vi "Periodic Tasks.vi"(8 "error in":errorcluster) -> ()   [LabVIEW 2013]
doc: "This VI runs in parallel to other tasks. It can contain as many user-defined periodic loops as you need. These can carry out PID or other sorts of timed response."
uses:
  <vilib>/Rock Robotics/SystemInterfaces/Utilities/FPGA_UtilitiesLED Source.ctl
  <vilib>/Rock Robotics/SystemInterfaces/Utilities/FPGA_UtilitiesLED State.ctl
  <vilib>/Rock Robotics/WPI/DriverStation/DriverStationLCD/WPI_DriverStationLCDLCDLine.ctl
  Robot Global Data.vi
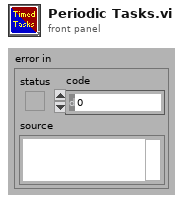
[diagram p1: front panel]
types:
  T1 = typedef "WPI_DigitalInputDevRef.ctl" = cluster{"DevStatus":errorcluster, "DIO Channel":T2, "Digital Module":T3}
  T2 = typedef "FPGA_DIOChannel.ctl" = enum8{"DIO 1", "DIO 2", "DIO 3", "DIO 4", "DIO 5", "DIO 6", "DIO 7", "DIO 8", "DIO 9", "DIO 10", "DIO 11", "DIO 12", "DIO 13", "DIO 14", "Invalid"}
  T3 = typedef "FPGA_TypedefDigitalModule.ctl" = enum16{"Digital Module 1", "Digital Module 2"}
  T4 = typedef "WPI_AnalogChannelDevRef.ctl" = cluster{"DevStatus":errorcluster, "Analog Module":T5, "Analog Channel":T6}
  T5 = typedef "FPGA_TypedefAnalogModule.ctl" = enum16{"Analog Module 1", "Analog Module 2"}
  T6 = typedef "FPGA_AIChannel.ctl" = enum8{"AI 1", "AI 2", "AI 3", "AI 4", "AI 5", "AI 6", "AI 7", "AI 8", "Invalid"}
  T7 = typedef "WPI_EncoderDevRef.ctl" = cluster{"DevStatus":errorcluster, "EncoderIndex":T8, "CounterIndex":T9, "DistancePerCount":dbl, "Decoding Type":T10}
  T8 = typedef "FPGA_EncoderIdx.ctl" = enum8{"Enc 0", "Enc 1", "Enc 2", "Enc 3", "Invalid"}
  T9 = typedef "FPGA_CounterCtrSystemIndex.ctl" = enum8{"Ctr 0", "Ctr 1", "Ctr 2", "Ctr 3", "Ctr 4", "Ctr 5", "Ctr 6", "Ctr 7", "Invalid"}
  T10 = typedef "WPI_EncoderType.ctl" = enum16{"1x", "2x", "4x"}
  T11 = cluster{"Winch Desired Location":dbl, "Winch Desired Location 2":dbl, "Winch Desired Location 3":dbl}
  T12 = typedef "FPGA_UtilitiesLED State.ctl" = enum16{"Off", "On", "Toggle"}
  T13 = typedef "FPGA_UtilitiesLED Source.ctl" = enum16{"User LED", "FPGA LED"}
  T14 = typedef "WPI_DriverStationLCDLCDLine.ctl" = enum16{"Main - Line 1", "User - Line 2", "User - Line 3", "User - Line 4", "User - Line 5", "User - Line 6"}
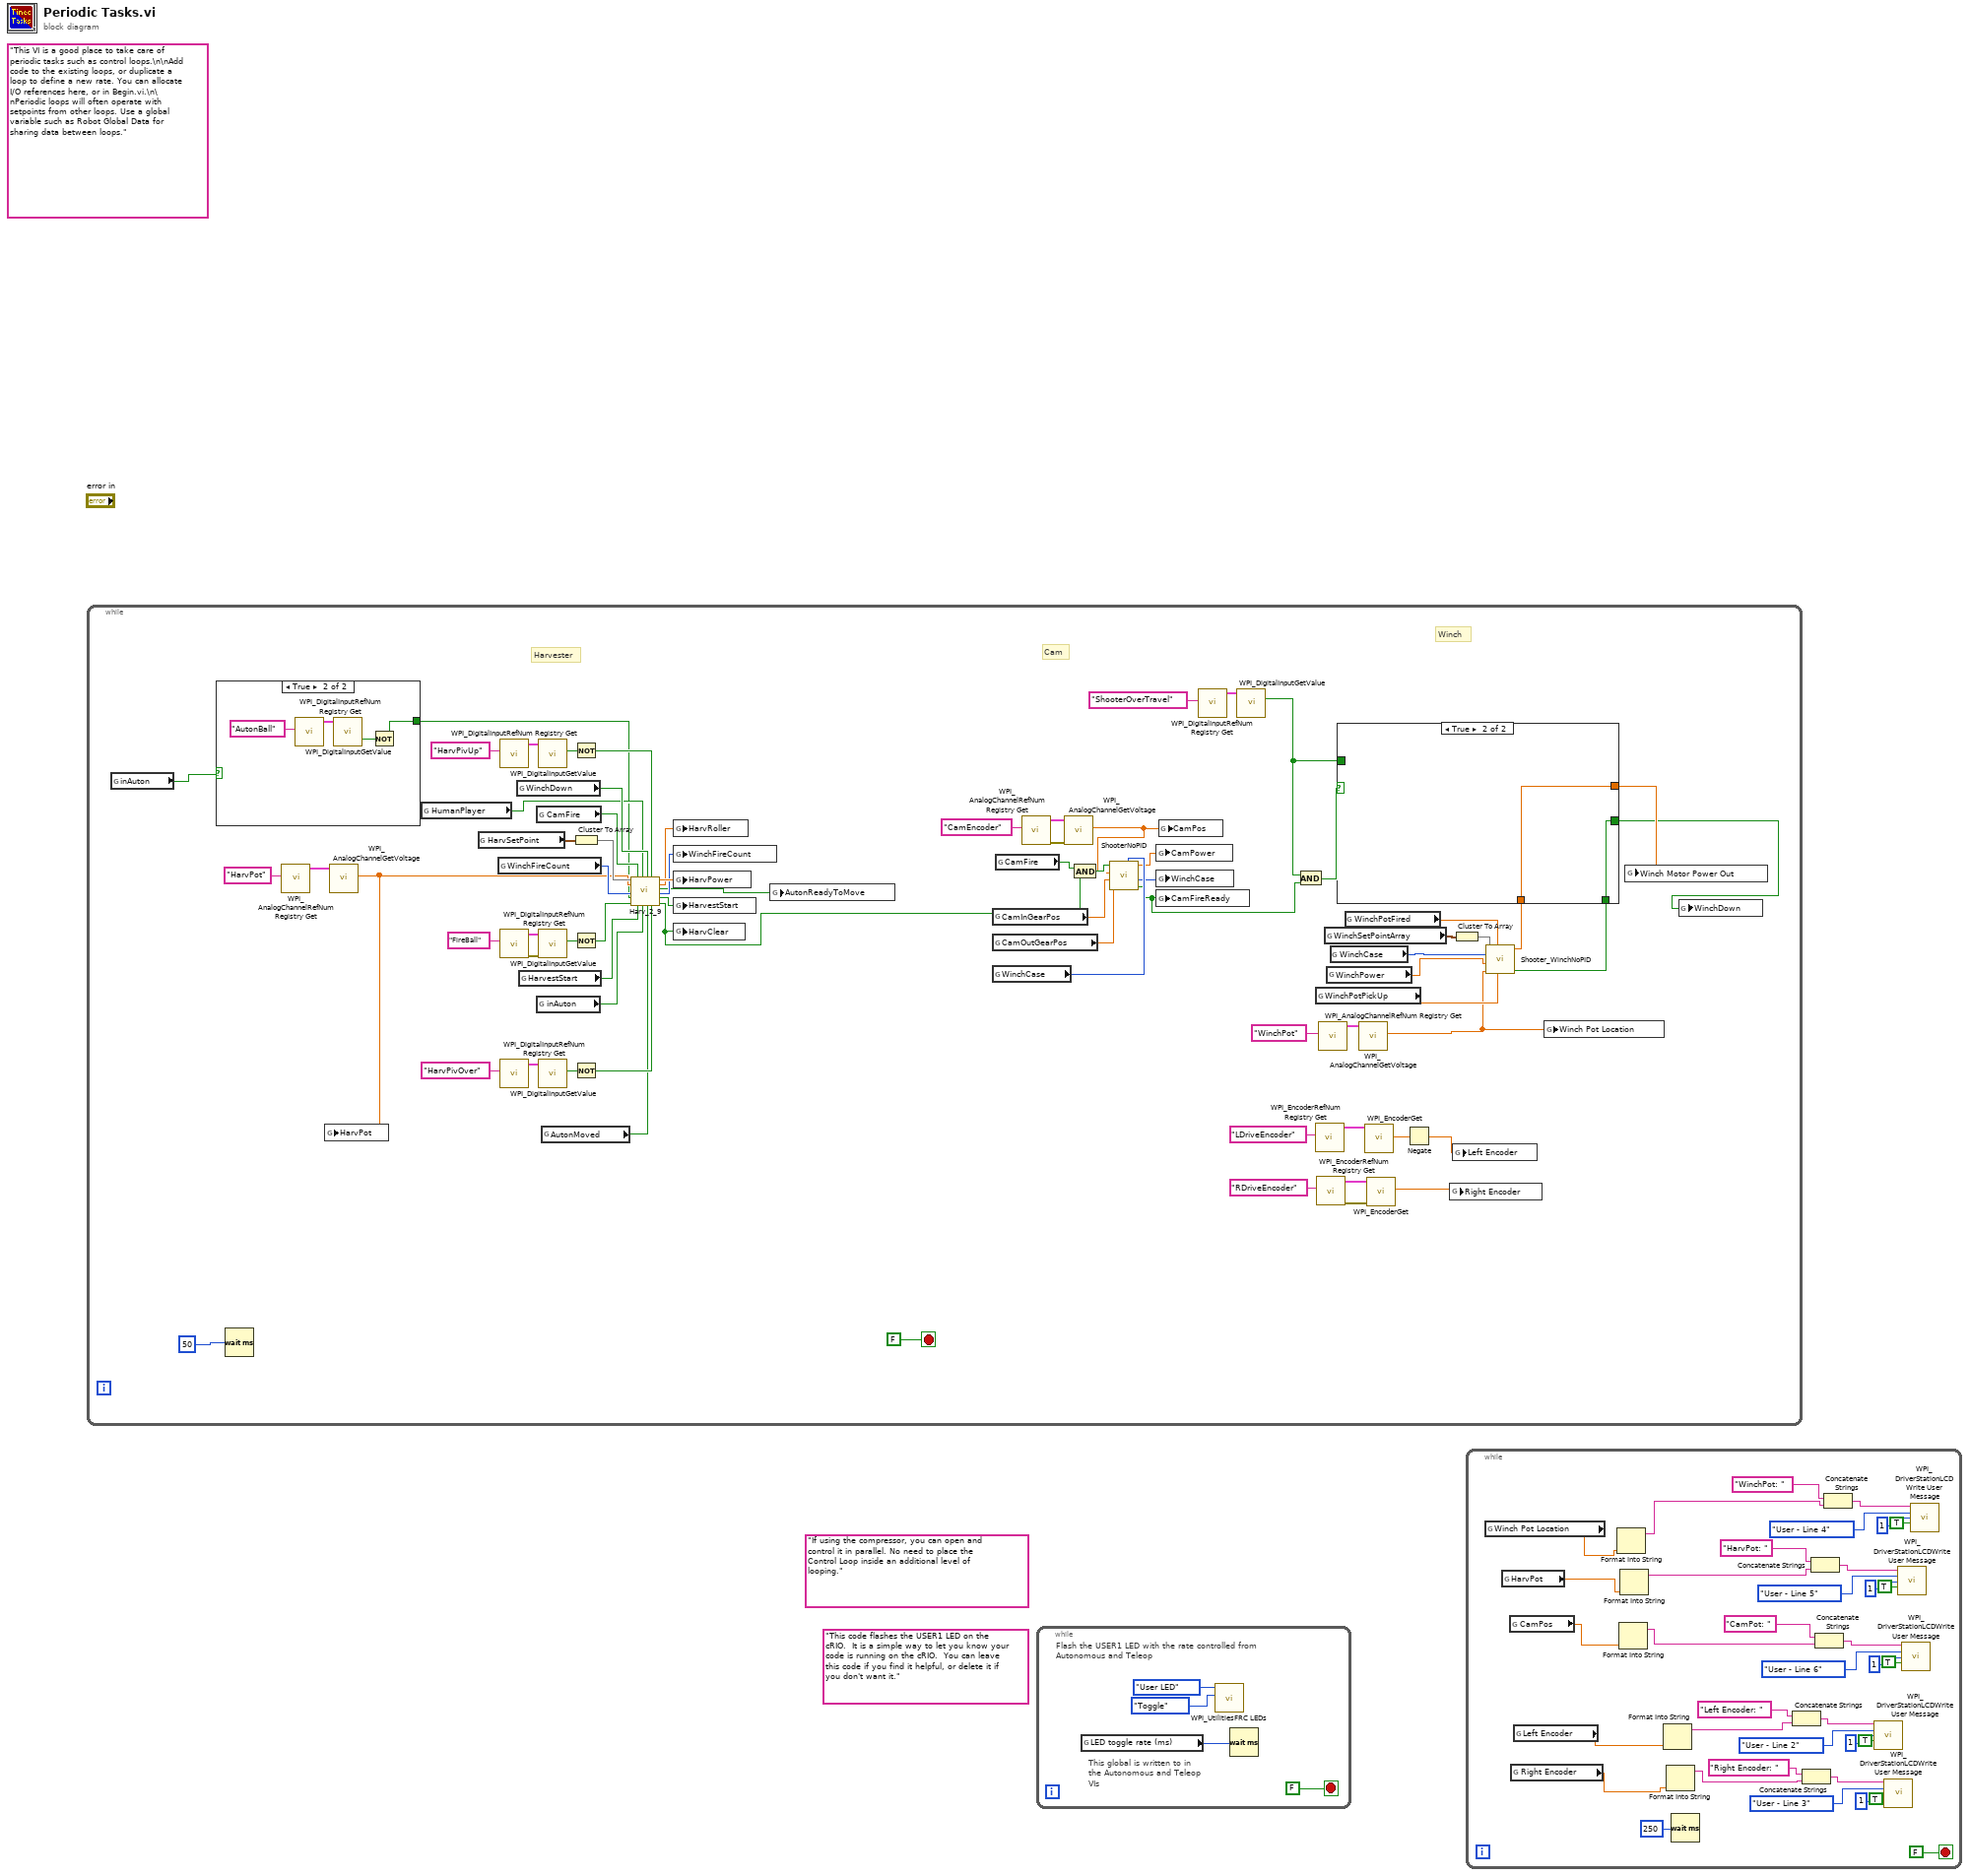
[diagram p0: block diagram]
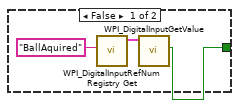
[diagram p2: hidden frame]
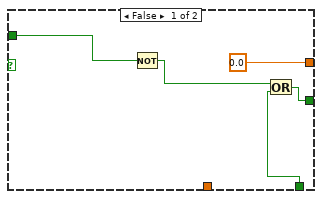
[diagram p3: hidden frame]
diagram:
  (unwired) "If using the compressor, you can open and control it in parallel. No need to place the Control Loop inside an additional level of looping."
  (unwired) "This code flashes the USER1 LED on the cRIO.  It is a simple way to let you know your code is running on the cRIO.  You can leave this code if you find it helpful, or delete it if you don't want it."
  (unwired) "This VI is a good place to take care of periodic tasks such as control loops.\n\nAdd code to the existing loops, or duplicate a loop to define a new rate. You can allocate I/O references here, or in Begin.vi.\n\nPeriodic loops will often operate with setpoints from other loops. Use a global variable such as Robot Global Data for sharing data between loops."
  n1 = while {
    stop <- FALSE stop-if-true
    # "Winch"
    # "Cam"
    # "Harvester"
    n2 = global read "Robot Global Data.vi" "inAuton"() -> (w2:bool)
    n3 = case shown="True" w2 {
      tunnel: [w73 w77] -> w1
      frame False {
        n4 = call <vilib>:"WPI_DigitalInputRefNum Registry Get.vi"("refnum name"="BallAquired") -> ("DigitalInputDevRef"=w75:T1)  [unwired: 9 in, 1 out]
        n5 = call <vilib>:"WPI_DigitalInputGetValue.vi"("DigitalInputDevRef"=w75) -> ("Value"=w73:bool)  [unwired: 8 in, 2 out]
      }
      frame True {
        n6 = call <vilib>:"WPI_DigitalInputRefNum Registry Get.vi"("refnum name"="AutonBall") -> ("DigitalInputDevRef"=w79:T1)  [unwired: 9 in, 1 out]
        n7 = call <vilib>:"WPI_DigitalInputGetValue.vi"("DigitalInputDevRef"=w79) -> ("Value"=w76:bool)  [unwired: 8 in, 2 out]
        n8 = Not(x=w76) -> (.not. x?=w77:bool)
      }
    }
    n9 = Wait (ms)(milliseconds to wait=u32 50) -> ()  [unwired: 1 out]
    n10 = call <vilib>:"WPI_AnalogChannelRefNum Registry Get.vi"("refnum name"="HarvPot") -> ("AIDeviceRef"=w71:T4)  [unwired: 9 in, 1 out]
    n11 = call <vilib>:"WPI_AnalogChannelGetVoltage.vi"("AIDeviceRef"=w71) -> ("Voltage"=w14:dbl)  [unwired: 8 in, 2 out]
    n12 = global write "Robot Global Data.vi" "HarvPot"(w14) -> ()
    n13 = global read "Robot Global Data.vi" "HumanPlayer"() -> (w5:bool)
    n14 = global read "Robot Global Data.vi" "HarvSetPoint"() -> (w42:cluster{"Out":dbl, "In":dbl, "Clear":dbl})
    n15 = global read "Robot Global Data.vi" "WinchFireCount"() -> (w17:i32)
    n16 = call <vilib>:"WPI_DigitalInputRefNum Registry Get.vi"("refnum name"="HarvPivUp") -> ("DigitalInputDevRef"=w55:T1)  [unwired: 9 in, 1 out]
    n17 = call <vilib>:"WPI_DigitalInputRefNum Registry Get.vi"("refnum name"="FireBall") -> ("error out"=w47:errorcluster, "DigitalInputDevRef"=w48:T1)  [unwired: 9 in]
    n18 = call <vilib>:"WPI_DigitalInputRefNum Registry Get.vi"("refnum name"="HarvPivOver") -> ("DigitalInputDevRef"=w63:T1)  [unwired: 9 in, 1 out]
    n19 = global read "Robot Global Data.vi" "WinchDown"() -> (w35:bool)
    n20 = global read "Robot Global Data.vi" "HarvestStart"() -> (w45:bool)
    n21 = global read "Robot Global Data.vi" "CamFire"() -> (w46:bool)
    n22 = global read "Robot Global Data.vi" "inAuton"() -> (w19:bool)
    n23 = call <vilib>:"WPI_DigitalInputGetValue.vi"("DigitalInputDevRef"=w55) -> ("Value"=w38:bool)  [unwired: 8 in, 2 out]
    n24 = call <vilib>:"WPI_DigitalInputGetValue.vi"("error in (no error)"=w47, "DigitalInputDevRef"=w48) -> ("Value"=w44:bool)  [unwired: 7 in, 2 out]
    n25 = call <vilib>:"WPI_DigitalInputGetValue.vi"("DigitalInputDevRef"=w63) -> ("Value"=w40:bool)  [unwired: 8 in, 2 out]
    n26 = global read "Robot Global Data.vi" "AutonMoved"() -> (w4:bool)
    n27 = Not(x=w38) -> (.not. x?=w37:bool)
    n28 = Cluster To Array(cluster=w42) -> (array=w41:dbl[])
    n29 = Not(x=w44) -> (.not. x?=w43:bool)
    n30 = Not(x=w40) -> (.not. x?=w39:bool)
    n31 = call "Harv_2_9.vi"("HarvSetpoints"=w41, "HarvPot"=w14, "Count"=w17, "BallAcquired"=w1, "FireBallSen"=w43, "Fire"=w46, "Harvest"=w45, "HPButton"=w5, "inAuton?"=w19, "WinchDown"=w35, "AutonMoved"=w4, "HarvPivUP"=w37, "HarvPivPickupLim"=w39) -> ("HarvPower"=w51:dbl, "HarvRoller"=w50:dbl, "AutonReadyToMove"=w3:bool, "CountOut"=w16:i32, "HarvStart"=w36:bool, "HarvCleared"=w9:bool)  [unwired: 1 in]
    n32 = global write "Robot Global Data.vi" "HarvRoller"(w50) -> ()
    n33 = global write "Robot Global Data.vi" "WinchFireCount"(w16) -> ()
    n34 = global write "Robot Global Data.vi" "HarvPower"(w51) -> ()
    n35 = global write "Robot Global Data.vi" "HarvestStart"(w36) -> ()
    n36 = global write "Robot Global Data.vi" "HarvClear"(w9) -> ()
    n37 = global write "Robot Global Data.vi" "AutonReadyToMove"(w3) -> ()
    n38 = global read "Robot Global Data.vi" "CamInGearPos"() -> (w24:dbl)
    n39 = global read "Robot Global Data.vi" "CamOutGearPos"() -> (w23:dbl)
    n40 = global read "Robot Global Data.vi" "WinchCase"() -> (w25:i32)
    n41 = global read "Robot Global Data.vi" "CamFire"() -> (w57:bool)
    n42 = call <vilib>:"WPI_AnalogChannelRefNum Registry Get.vi"("refnum name"="CamEncoder") -> ("error out"=w59:errorcluster, "AIDeviceRef"=w58:T4)  [unwired: 9 in]
    n43 = call <vilib>:"WPI_AnalogChannelGetVoltage.vi"("error in (no error)"=w59, "AIDeviceRef"=w58) -> ("Voltage"=w13:dbl)  [unwired: 7 in, 2 out]
    n44 = And(x=w57, y=w9) -> (x .and. y?=w26:bool)
    n45 = call "ShooterNoPID.vi"("WinchCaseIn"=w25, "InGearPosLow"=w23, "InGearPosHigh"=w24, "Pot"=w13, "Fire"=w26) -> ("There?"=w20:bool, "WinchCase"=w21:i32, "Power"=w22:dbl)  [unwired: 4 in]
    n46 = global write "Robot Global Data.vi" "CamPower"(w22) -> ()
    n47 = global write "Robot Global Data.vi" "WinchCase"(w21) -> ()
    n48 = global write "Robot Global Data.vi" "CamFireReady"(w20) -> ()
    n49 = global write "Robot Global Data.vi" "CamPos"(w13) -> ()
    n50 = call <vilib>:"WPI_DigitalInputRefNum Registry Get.vi"("refnum name"="ShooterOverTravel") -> ("DigitalInputDevRef"=w54:T1)  [unwired: 9 in, 1 out]
    n51 = call <vilib>:"WPI_DigitalInputGetValue.vi"("DigitalInputDevRef"=w54) -> ("Value"=w34:bool)  [unwired: 8 in, 2 out]
    n52 = And(x=w34, y=w20) -> (x .and. y?=w52:bool)
    n53 = global read "Robot Global Data.vi" "WinchPotPickUp"() -> (w18:dbl)
    n54 = call <vilib>:"WPI_EncoderRefNum Registry Get.vi"("refnum name"="LDriveEncoder") -> ("EncoderDevRef"=w65:T7)  [unwired: 9 in, 1 out]
    n55 = call <vilib>:"WPI_EncoderRefNum Registry Get.vi"("refnum name"="RDriveEncoder") -> ("error out"=w12:errorcluster, "EncoderDevRef"=w11:T7)  [unwired: 9 in]
    n56 = call <vilib>:"WPI_AnalogChannelRefNum Registry Get.vi"("refnum name"="WinchPot") -> ("AIDeviceRef"=w67:T4)  [unwired: 9 in, 1 out]
    n57 = global read "Robot Global Data.vi" "WinchSetPointArray"() -> (w31:T11)
    n58 = global read "Robot Global Data.vi" "WinchPower"() -> (w33:dbl)
    n59 = global read "Robot Global Data.vi" "WinchCase"() -> (w30:i32)
    n60 = global read "Robot Global Data.vi" "WinchPotFired"() -> (w6:dbl)
    n61 = call <vilib>:"WPI_AnalogChannelGetVoltage.vi"("AIDeviceRef"=w67) -> ("Voltage"=w15:dbl)  [unwired: 8 in, 2 out]
    n62 = call <vilib>:"WPI_EncoderGet.vi"("EncoderDevRef"=w65) -> ("Distance"=w8:dbl)  [unwired: 5 in, 5 out]
    n63 = call <vilib>:"WPI_EncoderGet.vi"("error in (no error)"=w12, "EncoderDevRef"=w11) -> ("Distance"=w10:dbl)  [unwired: 4 in, 5 out]
    n64 = Negate(x=w8) -> (-x=w7:dbl)
    n65 = global write "Robot Global Data.vi" "Right Encoder"(w10) -> ()
    n66 = Cluster To Array(cluster=w31) -> (array=w32:dbl[])
    n67 = global write "Robot Global Data.vi" "Left Encoder"(w7) -> ()
    n68 = call "Shooter_WinchNoPID.vi"("PickStartPos"=w18, "WinchFiredPos"=w6, "Winch Pot Location"=w15, "WinchPower"=w33, "selectedCase"=w30, "SetPointArray"=w32) -> ("isThere?"=w28:bool, "Winch Motor Power Out"=w27:dbl)  [unwired: 4 in]
    n69 = case shown="True" w52 {
      tunnel: [0.0 ("Winch Motor Power Out") w85] -> w61
      tunnel: [w83 w86] -> w29
      tunnel: w34 -> [w82 _]
      tunnel: w28 -> [w80 w86]
      tunnel: w27 -> [_ w85]
      frame False {
        n70 = Not(x=w82) -> (.not. x?=w81:bool)
        n71 = Or(x=w81, y=w80) -> (x .or. y?=w83:bool)
      }
      frame True {
      }
    }
    n72 = global write "Robot Global Data.vi" "Winch Pot Location"(w15) -> ()
    n73 = global write "Robot Global Data.vi" "Winch Motor Power Out"(w61) -> ()
    n74 = global write "Robot Global Data.vi" "WinchDown"(w29) -> ()
  }
  n75 = while {
    stop <- FALSE stop-if-true
    # "This global is written to in the Autonomous and Teleop VIs"
    # "Flash the USER1 LED with the rate controlled from Autonomous and Teleop"
    n76 = global read "Robot Global Data.vi" "LED toggle rate (ms)"() -> (w87:u32)
    n77 = call <vilib>:"WPI_UtilitiesFRC LEDs.vi"("State"=FPGA_UtilitiesLED_State."Toggle", "LED Type"=FPGA_UtilitiesLED_Source."User LED") -> ()  [unwired: 1 in, 9 out]
    n78 = Wait (ms)(milliseconds to wait=w87) -> ()  [unwired: 1 out]
  }
  n79 = while {
    stop <- FALSE stop-if-true
    n80 = global read "Robot Global Data.vi" "Winch Pot Location"() -> (w96:dbl)
    n81 = global read "Robot Global Data.vi" "HarvPot"() -> (w95:dbl)
    n82 = global read "Robot Global Data.vi" "CamPos"() -> (w97:dbl)
    n83 = global read "Robot Global Data.vi" "Right Encoder"() -> (w93:dbl)
    n84 = global read "Robot Global Data.vi" "Left Encoder"() -> (w94:dbl)
    n85 = Format Into String(w96) -> (resulting string=w113:string)  [unwired: 3 in, 1 out]
    n86 = Format Into String(w97) -> (resulting string=w98:string)  [unwired: 3 in, 1 out]
    n87 = Format Into String(w95) -> (resulting string=w107:string)  [unwired: 3 in, 1 out]
    n88 = Format Into String(w94) -> (resulting string=w105:string)  [unwired: 3 in, 1 out]
    n89 = Format Into String(w93) -> (resulting string=w104:string)  [unwired: 3 in, 1 out]
    n90 = Wait (ms)(milliseconds to wait=u32 250) -> ()  [unwired: 1 out]
    n91 = Concatenate Strings("Left Encoder: ", w105) -> (w123:string)
    n92 = Concatenate Strings("Right Encoder: ", w104) -> (w122:string)
    n93 = Concatenate Strings("HarvPot: ", w107) -> (w108:string)
    n94 = Concatenate Strings("CamPot: ", w98) -> (w103:string)
    n95 = Concatenate Strings("WinchPot: ", w113) -> (w118:string)
    n96 = call <vilib>:"WPI_DriverStationLCDWrite User Message.vi"("line text"=w123, "line"=WPI_DriverStationLCDLCDLine."User - Line 2", "starting column"=i8 1, "clear line before write (T)"=TRUE) -> ()  [unwired: 1 in, 11 out]
    n97 = call <vilib>:"WPI_DriverStationLCDWrite User Message.vi"("line text"=w122, "line"=WPI_DriverStationLCDLCDLine."User - Line 3", "starting column"=i8 1, "clear line before write (T)"=TRUE) -> ()  [unwired: 1 in, 11 out]
    n98 = call <vilib>:"WPI_DriverStationLCDWrite User Message.vi"("line text"=w108, "line"=WPI_DriverStationLCDLCDLine."User - Line 5", "starting column"=i8 1, "clear line before write (T)"=TRUE) -> ()  [unwired: 1 in, 11 out]
    n99 = call <vilib>:"WPI_DriverStationLCDWrite User Message.vi"("line text"=w103, "line"=WPI_DriverStationLCDLCDLine."User - Line 6", "starting column"=i8 1, "clear line before write (T)"=TRUE) -> ()  [unwired: 1 in, 11 out]
    n100 = call <vilib>:"WPI_DriverStationLCDWrite User Message.vi"("line text"=w118, "line"=WPI_DriverStationLCDLCDLine."User - Line 4", "starting column"=i8 1, "clear line before write (T)"=TRUE) -> ()  [unwired: 1 in, 11 out]
  }
